vi "UHR-Fleezers Control (host) -Leonardo 04-2018 V3.vi"(0 "Tab Control":T5(tab)=enum."Trap Control (RF)") -> ()   [LabVIEW 2013] (continued)
      tunnel: w2352 -> [_ w2837]
      tunnel: w2351 -> [_ w2810]
      frame False {
      }
      frame True {
        w2817 = u32 0 items=["Horizontal", "Vertical", "Central", "1st Diagonal", "2nd Diagonal"] ("Type of Symmetry")
        w2845 = u32 0 items=["Horizontal", "Vertical", "Central", "1st Diagonal", "2nd Diagonal"] ("Type of Symmetry")
        w2848 = u32 0 items=["Horizontal", "Vertical", "Central", "1st Diagonal", "2nd Diagonal"] ("Type of Symmetry")
        w2877 = u32 0 items=["Horizontal", "Vertical", "Central", "1st Diagonal", "2nd Diagonal"] ("Type of Symmetry")
        n1850 = Index Array(array=w2906, index=10) -> (element=w2912:waveform(dbl))
        n1851 = Index Array(array=w2906, index=11) -> (element=w2909:waveform(dbl))
        n1852 = local read "Cycles/step (MCL)"() -> (w2862:u64)
        n1853 = Index Array(array=w2906, index="Channel") -> (element=w2908:waveform(dbl))
        n1854 = Unbundle(w2810) -> ("New Image"=w2809:T3, "New Image"=w2808:T3, "New Image"=w2807:T3, "New Image"=w2806:T3)
        n1855 = Unbundle By Name(w2912) -> ("Y"=w2864:dbl[])
        n1856 = Unbundle By Name(w2909) -> ("Y"=w2866:dbl[])
        n1857 = Unbundle By Name(w2908) -> ("Y"=w2871:dbl[])
        n1858 = call "downsample 1D array - double.vi"("Ave N"=w2862, "Array In"=w2864) -> ("Array Out"=w2863:dbl[])  [unwired: 1 out]
        n1859 = call "downsample 1D array - double.vi"("Ave N"=w2862, "Array In"=w2866) -> ("Array Out"=w2865:dbl[])  [unwired: 1 out]
        n1860 = call "downsample 1D array - double.vi"("Ave N"=w2862, "Array In"=w2871) -> ("Array Out"=w2870:dbl[])  [unwired: 1 out]
        n1861 = feedback #12(w2932) -> (w2933:dbl[])
        n1862 = Build Array (concatenate)(w2933, w2932) -> (w2914:dbl[])
        n1863 = feedback #13(w2837) -> (w2839:dbl[])
        n1864 = Build Array (concatenate)(w2839, w2837) -> (w2838:dbl[])
        n1865 = local read "Scan steps (MCL)"() -> (w2819:u64)
        n1866 = Select(t=w2932, s=w2836, f=w2914) -> (s? t:f=w2918:dbl[])
        n1867 = feedback-in #12(w2918) -> ()
        n1868 = Select(t=w2837, s=w2836, f=w2838) -> (s? t:f=w2820:dbl[])
        n1869 = feedback-in #13(w2820) -> ()
        n1870 = local read "Scan lines (y)"() -> (w2805:u64)
        n1871 = local read "N APD Samp/step"() -> (w2821:dbl)
        n1872 = feedback #14(w2863) -> (w2920:dbl[])
        n1873 = Build Array (concatenate)(w2920, w2863) -> (w2911:dbl[])
        n1874 = feedback #15(w2870) -> (w2930:dbl[])
        n1875 = Build Array (concatenate)(w2930, w2870) -> (w2929:dbl[])
        n1876 = feedback #16(w2865) -> (w2922:dbl[])
        n1877 = Build Array (concatenate)(w2922, w2865) -> (w2923:dbl[])
        n1878 = Select(t=w2863, s=w2836, f=w2911) -> (s? t:f=w2867:dbl[])
        n1879 = feedback-in #14(w2867) -> ()
        n1880 = Select(t=w2870, s=w2836, f=w2929) -> (s? t:f=w2869:dbl[])
        n1881 = feedback-in #15(w2869) -> ()
        n1882 = Select(t=w2865, s=w2836, f=w2923) -> (s? t:f=w2868:dbl[])
        n1883 = feedback-in #16(w2868) -> ()
        n1884 = Multiply(x=w2819, y=u64 2) -> (x*y=w2804:u64)
        n1885 = call "integrate 1D array interval - double.vi"("Ave N"=w2821, "Array In"=w2820) -> ("Array Out"=w2832:dbl[])  [unwired: 1 out]
        n1886 = call "integrate 1D array interval - double.vi"("Ave N"=w2821, "Array In"=w2918) -> ("Array Out"=w2917:dbl[])  [unwired: 1 out]
        n1887 = Array Size(array=w2832) -> (size(s)=w2833:i32)
        n1888 = Array Size(array=w2917) -> (size(s)=w2919:i32)
        n1889 = Multiply(x=w2805, y=w2804) -> (x*y=w2835:u64)
        n1890 = Multiply(x=w2805, y=w2804) -> (x*y=w2927:u64)
        n1891 = call-poly <vilib>:"Mean.vi"("X"=w2867) -> ("mean"=w2851:dbl)  [unwired: 1 out]
        n1892 = Subtract(x=w2835, y=w2833) -> (x-y=w2826:u64)
        n1893 = call-poly <vilib>:"Mean.vi"("X"=w2869) -> ("mean"=w2856:dbl)  [unwired: 1 out]
        n1894 = call-poly <vilib>:"Mean.vi"("X"=w2868) -> ("mean"=w2854:dbl)  [unwired: 1 out]
        n1895 = call-poly <vilib>:"Mean.vi"("X"=w2832) -> ("mean"=w2823:dbl)  [unwired: 1 out]
        n1896 = Subtract(x=w2927, y=w2919) -> (x-y=w2861:u64)
        n1897 = call-poly <vilib>:"Mean.vi"("X"=w2917) -> ("mean"=w2858:dbl)  [unwired: 1 out]
        n1898 = Initialize Array(1.0 ("element"), w2826) -> (w2822:dbl[])
        n1899 = Initialize Array(1.0 ("element"), w2861) -> (w2852:dbl[])
        n1900 = Multiply(x=w2822, y=w2823) -> (x*y=w2824:dbl[])
        n1901 = Multiply(x=w2852, y=w2854) -> (x*y=w2855:dbl[])
        n1902 = Multiply(x=w2852, y=w2856) -> (x*y=w2857:dbl[])
        n1903 = Multiply(x=w2852, y=w2851) -> (x*y=w2853:dbl[])
        n1904 = Multiply(x=w2852, y=w2858) -> (x*y=w2859:dbl[])
        n1905 = Build Array (concatenate)(w2867, w2853) -> (w2921:dbl[])
        n1906 = Build Array (concatenate)(w2869, w2857) -> (w2925:dbl[])
        n1907 = Build Array (concatenate)(w2868, w2855) -> (w2924:dbl[])
        n1908 = Build Array (concatenate)(w2832, w2824) -> (w2834:dbl[])
        n1909 = Build Array (concatenate)(w2917, w2859) -> (w2926:dbl[])
        n1910 = Reshape Array(w2921, w2805, w2804) -> (w2887:dbl[][])
        n1911 = Reshape Array(w2834, w2805, w2804) -> (w2830:dbl[][])
        n1912 = Reshape Array(w2925, w2805, w2804) -> (w2879:dbl[][])
        n1913 = Reshape Array(w2924, w2805, w2804) -> (w2894:dbl[][])
        n1914 = Reshape Array(w2926, w2805, w2804) -> (w2904:dbl[][])
        n1915 = Array Subset(array=w2894, index (col)=0 ("index"), length (col)=w2819) -> (w2899:dbl[][])  [unwired: 2 in]
        n1916 = Array Subset(array=w2894, index (col)=w2819) -> (w2897:dbl[][])  [unwired: 3 in]
        n1917 = Array Subset(array=w2879, index (col)=0 ("index"), length (col)=w2819) -> (w2885:dbl[][])  [unwired: 2 in]
        n1918 = Array Subset(array=w2879, index (col)=w2819) -> (w2883:dbl[][])  [unwired: 3 in]
        n1919 = Array Subset(array=w2830, index (col)=0 ("index"), length (col)=w2819) -> (w2829:dbl[][])  [unwired: 2 in]
        n1920 = Array Subset(array=w2830, index (col)=w2819) -> (w2827:dbl[][])  [unwired: 3 in]
        n1921 = Array Subset(array=w2904, index (col)=0 ("index"), length (col)=w2819) -> (w2903:dbl[][])  [unwired: 2 in]
        n1922 = Array Subset(array=w2904, index (col)=w2819) -> (w2901:dbl[][])  [unwired: 3 in]
        n1923 = Array Subset(array=w2887, index (col)=0 ("index"), length (col)=w2819) -> (w2892:dbl[][])  [unwired: 2 in]
        n1924 = Array Subset(array=w2887, index (col)=w2819) -> (w2890:dbl[][])  [unwired: 3 in]
        n1925 = for {
          tunnel: w2899 -> [w2941] mode=indexing
          tunnel: [w2940] -> w2898 mode=indexing
          workers-P: _ -> [_]
          n1926 = Reverse 1D Array(array=w2941) -> (reversed array=w2940:dbl[])
        }
        n1927 = for {
          tunnel: w2885 -> [w2937] mode=indexing
          tunnel: [w2936] -> w2884 mode=indexing
          workers-P: _ -> [_]
          n1928 = Reverse 1D Array(array=w2937) -> (reversed array=w2936:dbl[])
        }
        n1929 = for {
          tunnel: w2829 -> [w2935] mode=indexing
          tunnel: [w2934] -> w2828 mode=indexing
          workers-P: _ -> [_]
          n1930 = Reverse 1D Array(array=w2935) -> (reversed array=w2934:dbl[])
        }
        n1931 = for {
          tunnel: w2903 -> [w2943] mode=indexing
          tunnel: [w2942] -> w2902 mode=indexing
          workers-P: _ -> [_]
          n1932 = Reverse 1D Array(array=w2943) -> (reversed array=w2942:dbl[])
        }
        n1933 = for {
          tunnel: w2892 -> [w2939] mode=indexing
          tunnel: [w2938] -> w2891 mode=indexing
          workers-P: _ -> [_]
          n1934 = Reverse 1D Array(array=w2939) -> (reversed array=w2938:dbl[])
        }
        n1935 = Index Array(array=w2904, index (row)=0) -> (element=→"Waveform Graph":dbl[])  [unwired: 1 in]
        n1936 = Add(x=w2898, y=w2897) -> (x+y=w2896:dbl[][])
        n1937 = Add(x=w2884, y=w2883) -> (x+y=w2882:dbl[][])
        n1938 = Add(x=w2828, y=w2827) -> (x+y=w2812:dbl[][])
        n1939 = Add(x=w2902, y=w2901) -> (x+y=w2876:dbl[][])
        n1940 = Add(x=w2891, y=w2890) -> (x+y=w2889:dbl[][])
        n1941 = Divide(x=w2882, y=2) -> (x/y=w2880:dbl[][])
        n1942 = Divide(x=w2896, y=2) -> (x/y=w2841:dbl[][])
        n1943 = Divide(x=w2889, y=2) -> (x/y=w2843:dbl[][])
        n1944 = To Single Precision Float(number=w2876) -> (single precision float=w2875:sgl[][])
        n1945 = Transpose 2D Array(2D array=w2880) -> (transposed array=→"Data map":dbl[][])
        n1946 = To Single Precision Float(number=w2812) -> (single precision float=w2816:sgl[][])
        n1947 = To Single Precision Float(number=w2841) -> (single precision float=w2847:sgl[][])
        n1948 = To Single Precision Float(number=w2843) -> (single precision float=w2844:sgl[][])
        n1949 = call "IMAQ ArrayToImage"("Image Pixels (Float)"=w2875, "Image"=w2809) -> ("Image Out"=w2878:T3)  [unwired: 8 in, 1 out]
        n1950 = call "IMAQ ArrayToImage"("Image Pixels (Float)"=w2816, "Image"=w2808) -> ("Image Out"=w2818:T3)  [unwired: 8 in, 1 out]
        n1951 = call "IMAQ ArrayToImage"("Image Pixels (Float)"=w2847, "Image"=w2807) -> ("Image Out"=w2849:T3)  [unwired: 8 in, 1 out]
        n1952 = call "IMAQ ArrayToImage"("Image Pixels (Float)"=w2844, "Image"=w2806) -> ("Image Out"=w2846:T3)  [unwired: 8 in, 1 out]
        n1953 = call "IMAQ Symmetry"("Type of Symmetry"=w2877, "Image Src"=w2878) -> ("Image Dst Out"=w2873:T3)  [unwired: 3 in, 1 out]
        n1954 = call "IMAQ Symmetry"("Type of Symmetry"=w2817, "Image Src"=w2818) -> ("Image Dst Out"=w2814:T3)  [unwired: 3 in, 1 out]
        n1955 = call "IMAQ Symmetry"("Type of Symmetry"=w2848, "Image Src"=w2849) -> ("Image Dst Out"=→"Detection Laser X":T3)  [unwired: 3 in, 1 out]
        n1956 = call "IMAQ Symmetry"("Type of Symmetry"=w2845, "Image Src"=w2846) -> ("Image Dst Out"=→"Detection Laser Y":T3)  [unwired: 3 in, 1 out]
        n1957 = call "IMAQ Set Simple Calibration"("Calibration Axis Info"=T37 {"Origin Pixel"={"X"=0.0, "Y"=0.0}, "Angle Relative to Horizontal (deg)"=0.0, "Axis Reference"=0}, "Grid Descriptor"=T38 {"X Step"=0.3, "Y Step"=0.3, "Unit"=enum."Undefined"}, "Image"=w2873) -> ("Calibrated Image"=→"APD 1":T3)  [unwired: 7 in, 1 out]
        n1958 = call "IMAQ Set Simple Calibration"("Calibration Axis Info"=T37 {"Origin Pixel"={"X"=0.0, "Y"=0.0}, "Angle Relative to Horizontal (deg)"=0.0, "Axis Reference"=0}, "Grid Descriptor"=T38 {"X Step"=0.3, "Y Step"=0.3, "Unit"=enum."Undefined"}, "Image"=w2814) -> ("Calibrated Image"=→"APD 2":T3)  [unwired: 7 in, 1 out]
      }
    }
    n1959 = Subtract(x=w2358, y="APD 2 Offset") -> (x-y=w2355:waveform(dbl))
    n1960 = Subtract(x=w2360, y="APD 1 Offset") -> (x-y=w2356:waveform(dbl))
    n1961 = Index Array(array=w2375, index=3) -> (element=w2434:waveform(dbl))
    n1962 = Index Array(array=w2375, index=6) -> (element=w2431:waveform(dbl))
    n1963 = Build Array(w2356, w2355) -> (→"APD Chart":waveform(dbl)[])
    n1964 = Array Size(array=w2424) -> (size(s)=w2472:i32)
    n1965 = call <vilib>:"Std Deviation and Variance.vi"("X"=w2368) -> ("standard deviation"=w2367:dbl)  [unwired: 1 in, 2 out]
    n1966 = Add Array Elements(numeric array=w2368) -> (sum=w2370:u32)
    n1967 = Add Array Elements(numeric array=w2424) -> (sum=w2482:u32)
    n1968 = call <vilib>:"Std Deviation and Variance.vi"("X"=w2424) -> ("standard deviation"=w2423:dbl)  [unwired: 1 in, 2 out]
    n1969 = Divide(x=w2367, y=w2366) -> (x/y=w2363:dbl)
    "Rate sigma (Hz) 2" <- w2363
    n1970 = Multiply(x=w2366, y=w2472) -> (x*y=w2369:dbl)
    "Int. Time (s)" <- w2369
    n1971 = Divide(x=w2370, y=w2369) -> (x/y=w2364:dbl)
    "APD 2 Rate (Hz)" <- w2364
    n1972 = Divide(x=w2482, y=w2369) -> (x/y=w2421:dbl)
    "APD 1 Rate (Hz)" <- w2421
    n1973 = Divide(x=w2423, y=w2366) -> (x/y=w2422:dbl)
    "Rate sigma (Hz)" <- w2422
    n1974 = Divide(x=w2363, y=w2364) -> (x/y=→"Sigma/Mean 2":dbl)
    n1975 = Divide(x=w2422, y=w2421) -> (x/y=→"Sigma/Mean":dbl)
    n1976 = case shown="2" "Calibration" {
      tunnel: "T1 alpha_x (nm/V)" -> [_ w2772 w2793]
      tunnel: "T1 kappa_x (pN/nm)" -> [_ _ w2783]
      tunnel: "T2 alpha_x (nm/V)" -> [_ w2771 w2791]
      tunnel: "T2 kappa_x (pN/nm)" -> [_ _ w2784]
      tunnel: w2434 -> [w2754 w2769 w2789]
      tunnel: w2431 -> [w2753 w2767 w2787]
      tunnel: [w2754 w2766 w2786] -> w2224
      tunnel: [w2753 w2765 w2785] -> w2230
      tunnel: ["T1 X (V)" ("Label.Text") "T1 X (nm)" ("Label.Text") "T1 X (pN)" ("Label.Text")] -> w2452
      tunnel: ["T2 X (V)" ("Label.Text") "T2 X (nm)" ("Label.Text") "T2 X (pN)" ("Label.Text")] -> w2451
      tunnel: ["Position (V)" ("Label.Text") "Position (nm)" ("Label.Text") "Force (pN)" ("Label.Text")] -> w2453
      tunnel: w2433 -> [_ w2757 w2776]
      tunnel: w2435 -> [_ w2760 w2778]
      tunnel: ["Mean (V)" ("Label.Text") "Mean (nm)" ("Label.Text") "Mean (pN)" ("Label.Text")] -> w2448
      tunnel: ["Difference (V)" ("Label.Text") "Difference (nm)" ("Label.Text") "Difference (pN)" ("Label.Text")] -> w2383
      frame 0, Default {
      }
      frame 1 {
        # "position"
        n1977 = Unbundle By Name(w2769) -> ("Y"=w2773:dbl[])
        n1978 = Unbundle By Name(w2767) -> ("Y"=w2758:dbl[])
        n1979 = Subtract(x=w2773, y=w2760) -> (x-y=w2761:dbl[])
        n1980 = Subtract(x=w2758, y=w2757) -> (x-y=w2759:dbl[])
        n1981 = Multiply(x=w2759, y=w2771) -> (x*y=w2768:dbl[])
        n1982 = Multiply(x=w2772, y=w2761) -> (x*y=w2770:dbl[])
        n1983 = Bundle By Name(cluster=w2767, "Y"=w2768) -> (w2765:waveform(dbl))
        n1984 = Bundle By Name(cluster=w2769, "Y"=w2770) -> (w2766:waveform(dbl))
      }
      frame 2 {
        # "force"
        n1985 = Unbundle By Name(w2789) -> ("Y"=w2794:dbl[])
        n1986 = Unbundle By Name(w2787) -> ("Y"=w2792:dbl[])
        n1987 = Subtract(x=w2792, y=w2776) -> (x-y=w2777:dbl[])
        n1988 = Subtract(x=w2794, y=w2778) -> (x-y=w2779:dbl[])
        n1989 = Compound Arithmetic op=MULTIPLY(w2777, w2791, w2784) -> (w2788:dbl[])
        n1990 = Compound Arithmetic op=MULTIPLY(w2783, w2793, w2779) -> (w2790:dbl[])
        n1991 = Bundle By Name(cluster=w2787, "Y"=w2788) -> (w2785:waveform(dbl))
        n1992 = Bundle By Name(cluster=w2789, "Y"=w2790) -> (w2786:waveform(dbl))
      }
    }
    n1993 = feedback-in #17("Calibration") -> ()
    n1994 = feedback #17(u16 1 ("Calibration")) -> (w2455:u16)
    n1995 = local read "Trap 2 Bead Size (nm)"() -> (w2263:dbl)
    n1996 = local read "Trap 1 Bead Size (nm)"() -> (w2262:dbl)
    n1997 = local read "AOM X Cal (nm/MHz)"() -> (w2260:dbl)
    n1998 = local read "Trap Delta (MHz)"() -> (w2259:dbl)
    n1999 = Not Equal?(x=w2455, y="Calibration") -> (x != y?=w2412:bool)
    n2000 = Multiply(x=w2260, y=w2259) -> (x*y=w2264:dbl)
    n2001 = Unbundle By Name(w2224) -> ("Y"=w2229:dbl[])
    n2002 = Unbundle By Name(w2230) -> ("Y"=w2228:dbl[])
    n2003 = Add(x=w2263, y=w2262) -> (x+y=w2266:dbl)
    n2004 = case shown="False" "Negate trap 2 force" {
      tunnel: [-1.0 1.0] -> w2441
      frame False {
      }
      frame True {
      }
    }
    n2005 = Unbundle By Name(w2434) -> ("Y"=w2437:dbl[])
    n2006 = Unbundle By Name(w2431) -> ("Y"=w2440:dbl[])
    n2007 = Divide(x=w2266, y=2.0) -> (x/y=w2261:dbl)
    n2008 = Subtract(x=w2229, y=w2228) -> (x-y=w2226:dbl[])
    n2009 = Subtract(x=w2437, y=w2435) -> (x-y=w2438:dbl[])
    n2010 = Subtract(x=w2440, y=w2433) -> (x-y=w2439:dbl[])
    n2011 = Divide(x=w2226, y=2.0) -> (x/y=w2225:dbl[])
    n2012 = Multiply(x=w2439, y="T2 alpha_x (nm/V)") -> (x*y=w2430:dbl[])
    n2013 = Multiply(x="T1 alpha_x (nm/V)", y=w2438) -> (x*y=w2429:dbl[])
    n2014 = Multiply(x=w2230, y=w2441) -> (x*y=w2442:waveform(dbl))
    n2015 = Bundle By Name(cluster=w2224, "Y"=w2225) -> (w2223:waveform(dbl))
    n2016 = case shown="True" "Read Lateness and Rel Phase" {
      tunnel: w2236 -> [w2720 w2742]
      tunnel: w2275 -> [w2721 w2741]
      tunnel: [w2720 w2740] -> w2427
      tunnel: [w2721 w2739] -> w2426
      frame False {
      }
      frame True {
        n2017 = xnode "Read/Write Control"("FPGA VI Reference In"=w2742, "error in"=w2741) -> ("FPGA VI Reference Out"=w2740:T20, "error out"=w2739:errorcluster, "GI Relative phase"=→"GI relative phase":i16, "Relative phase"=→"Relative phase (AI1)":i16, "AI Late Counter"=→"Late Counter (AI1)":u8, "GI Late Counter"=→"GI Late Counter":u8, "MCL Late Counter"=→"MCL Late Counter":u8, "MCL Relative Phase"=→"Relative Phase (MCL)":i16, "APD Acq Relative Phase"=→"APD Acq Relative Phase":i16, "APD 1 Gate Relative Phase"=→"APD 1 Gate Relative Phase":i16, "APD 2 Gate Relative Phase"=→"APD 2 Gate Relative Phase":i16, "APD Acq Late Counter"=→"APD Acq Late Counter":u16, "APD 1 Gate Late Counter"=→"APD 1 Gate Late Counter":u8, "APD 2 Gate Late Counter"=→"APD 2 Gate Late Counter":u8, "Green FB Relative Phase"=→"Relative phase (Green FB)":i16, "GI Relative phase"=→"GI relative phase 2":i16, "GI Late Counter 2"=→"GI Late Counter 2":u16, "Trap Pos FIFO Timeout"=→"Trap Pos FIFO Timeout":u16, "Trap AI FIFO Timeout"=→"Trap AI FIFO Timeout":u16)
      }
    }
    n2018 = Subtract(x=w2430, y=w2429) -> (x-y=w2258:dbl[])
    n2019 = call-poly <vilib>:"Mean.vi"("X"=w2258) -> ("mean"=w2265:dbl)  [unwired: 1 out]
    n2020 = Add(x=w2264, y=w2265) -> (x+y=w2268:dbl)
    n2021 = Subtract(x=w2268, y=w2261) -> (x-y=→"Tether Extension (nm, calculated)":dbl)
    n2022 = Unbundle By Name(w2230) -> ("Y"=w2221:dbl[])
    n2023 = Unbundle By Name(w2224) -> ("Y"=w2222:dbl[])
    n2024 = Build Array(w2224, w2442, w2223) -> (→"Force":waveform(dbl)[])
    n2025 = Subtract(x=w2258, y="Offset (nm)") -> (x-y=w2402:dbl[])
    n2026 = call-poly <vilib>:"Mean.vi"("X"=w2221) -> ("mean"=w2219:dbl)  [unwired: 1 out]
    "T2 X" <- w2219
    n2027 = call-poly <vilib>:"Mean.vi"("X"=w2222) -> ("mean"=w2220:dbl)  [unwired: 1 out]
    "T1 X" <- w2220
    n2028 = Subtract(x=w2222, y=w2221) -> (x-y=w2404:dbl[])
    n2029 = Bundle By Name(cluster=w2434, "Y"=w2402) -> (w2374:waveform(dbl))
    "Bead Separation" <- w2374
    n2030 = Divide(x=w2404, y=2.0) -> (x/y=→"Vec Mean of T1 T2":dbl[])
    n2031 = case shown="True" w2412 {
      tunnel: w2453 -> [_ w2747]
      tunnel: w2452 -> [_ w2746]
      tunnel: w2451 -> [_ w2745]
      tunnel: w2448 -> [_ w2744]
      tunnel: w2383 -> [_ w2743]
      frame False {
      }
      frame True {
        n2032 = property on="Force" class="WFChart (strict)"("YScale.NameLbl.Text"=w2747) -> ()  [unwired: 2 in, 2 out]
        n2033 = property on="T2 X" class="DigNum (strict)"("Caption.Text"=w2745) -> ()  [unwired: 2 in, 2 out]
        n2034 = property on="T1 X" class="DigNum (strict)"("Caption.Text"=w2746) -> ()  [unwired: 2 in, 2 out]
        n2035 = property on="Mean" class="DigNum (strict)"("Caption.Text"=w2744) -> ()  [unwired: 2 in, 2 out]
        n2036 = property on="Difference" class="DigNum (strict)"("Caption.Text"=w2743) -> ()  [unwired: 2 in, 2 out]
      }
    }
    n2037 = local read "Tether"() -> (w2406:bool)
    n2038 = Subtract(x=w2220, y=w2219) -> (x-y=w2450:dbl)
    n2039 = Add(x=w2220, y=w2219) -> (x+y=→"Difference":dbl)
    n2040 = feedback #18(w2402) -> (w2401:dbl[])
    n2041 = Divide(x=w2450, y=2.0) -> (x/y=w2233:dbl)
    "Mean" <- w2233
    n2042 = case shown="True" w2406 {
      tunnel: w2233 -> [_ w2679]
      frame False {
      }
      frame True {
        n2043 = Greater?(x="Lost Tether Alarm Threshold (pN)", y=w2679) -> (0:w2677:bool)
        n2044 = case shown="True" w2677 {
          frame False {
          }
          frame True {
            n2045 = flat-sequence {
              frame #0 {
                # "stop only if saving"
                n2046 = local read "Saving..."() -> (w2692:bool)
                n2047 = And(x=w2692, y="TA Cancel Save?") -> (x .and. y?=w2691:bool)
                n2048 = local write "Stop Saving"(w2691) -> ()
              }
              frame #1 {
                n2049 = case shown="True" "TA Green Off?" {
                  frame False {
                  }
                  frame True {
                    w2695 = FALSE ("Fl. Triggered...")
                    n2050 = local write "Fl. Triggered..."(w2695) -> ()
                    n2051 = property on="Green Laser ON/Interlacing" class="Bool (strict)"("Val(Sgnl)"=w2695) -> ()  [unwired: 2 in, 2 out]
                  }
                }
              }
            }
            n2052 = local read "Time tether formed"() -> (w2686:timestamp)
            n2053 = Get Date/Time In Seconds() -> (seconds since 1Jan1904=w2687:timestamp)
            n2054 = Subtract(x=w2687, y=w2686) -> (x-y=w2685:dbl)
            n2055 = Number To Decimal String(number=w2685) -> (decimal integer string=w2682:string)  [unwired: 1 out]
            n2056 = local read "Messages"() -> (w2689:string)
            n2057 = call <vilib>:"Beep.vi"() -> ()  [unwired: 3 in, 9 out]
            n2058 = Concatenate Strings("Lost tether (" ("Message to add"), w2682, " s)." ("string")) -> (w2684:string)
            n2059 = local write "Tether"(FALSE ("Tether")) -> ()
            n2060 = call "Update messages.vi"("Message to add"=w2684, "Old message string"=w2689) -> ("New message string"=w2688:string)
            n2061 = local write "Messages"(w2688) -> ()
            n2062 = property on="Trap Pos. FB ON" class="Bool (strict)"("Val(Sgnl)"=FALSE ("Value (Signaling)")) -> ()  [unwired: 2 in, 2 out]
          }
        }
      }
    }
    n2063 = Build Array (concatenate)(w2402, w2401) -> (w2400:dbl[])
    n2064 = Split 1D Array(array=w2400, index=w2286) -> (first subarray=w2396:dbl[])  [unwired: 1 out]
    n2065 = feedback-in #18(w2396) -> ()
    n2066 = call-poly <vilib>:"Mean.vi"("X"=w2396) -> ("mean"=w2395:dbl)  [unwired: 1 out]
    "Bead Mean (nm)" <- w2395
    n2067 = Subtract(x=w2396, y=w2395) -> (x-y=w2394:dbl[])
    n2068 = Square(x=w2394) -> (x^2=w2393:dbl[])
    n2069 = case shown="True" "Semi Passive ON" {
      tunnel: "Semi Passive mode" -> [_ w2560]
      tunnel: "Jump Force (pN)" -> [_ w2559]
      tunnel: w2233 -> [_ w2558]
      frame False {
      }
      frame True {
        n2070 = case shown="\"Use Feedback\"" w2560 {
          tunnel: w2559 -> [_ w2563 w2579]
          tunnel: w2558 -> [_ w2562 w2578]
          frame "None" {
          }
          frame "Use Feedback" {
            n2071 = local read "Target Force (pN)"() -> (w2565:dbl)
            n2072 = Less?(x=w2563, y=w2565) -> (x < y?=w2564:bool)
            n2073 = case shown="True" w2564 {
              tunnel: w2563 -> [w2572 w2575]
              tunnel: w2562 -> [w2571 w2574]
              tunnel: [w2570 w2573] -> w2561
              frame False {
                n2074 = Less?(x=w2572, y=w2571) -> (x < y?=w2570:bool)
              }
              frame True {
                n2075 = Greater?(x=w2575, y=w2574) -> (0:w2573:bool)
              }
            }
            n2076 = case shown="True" w2561 {
              frame False {
                n2077 = local read "Trap Pos. FB ON"() -> (w2566:bool)
                n2078 = case shown="True" w2566 {
                  frame False {
                  }
                  frame True {
                    n2079 = property on="Trap Pos. FB ON" class="Bool (strict)"("Val(Sgnl)"=FALSE) -> ()  [unwired: 2 in, 2 out]
                  }
                }
              }
              frame True {
                n2080 = local read "Trap Pos. FB ON"() -> (w2568:bool)
                n2081 = case shown="False" w2568 {
                  frame False {
                    n2082 = property on="Trap Pos. FB ON" class="Bool (strict)"("Val(Sgnl)"=TRUE) -> ()  [unwired: 2 in, 2 out]
                  }
                  frame True {
                  }
                }
              }
            }
          }
          frame "Sharp Jump" {
            n2083 = local read "Target Force (pN)"() -> (w2581:dbl)
            n2084 = Greater?(x=w2579, y=w2581) -> (0:w2580:bool)
            n2085 = case shown="True" w2580 {
              tunnel: w2579 -> [w2596 w2600]
              tunnel: w2578 -> [w2597 w2599]
              tunnel: [w2595 w2598] -> w2577
              frame False {
                n2086 = Greater?(x=w2597, y=w2596) -> (0:w2595:bool)
              }
              frame True {
                n2087 = Less?(x=w2600, y=w2599) -> (x < y?=w2598:bool)
              }
            }
            n2088 = Subtract(x=w2579, y=w2581) -> (x-y=w2576:dbl)
            n2089 = case shown="True" w2577 {
              tunnel: w2576 -> [_ w2587]
              frame False {
              }
              frame True {
                n2090 = local read "T1 kappa_x (pN/nm)"() -> (w2592:dbl)
                n2091 = local read "T2 kappa_x (pN/nm)"() -> (w2593:dbl)
                n2092 = Reciprocal(x="DNA stiffness (pN / nm)") -> (1/x=w2589:dbl)
                n2093 = Reciprocal(x=w2592) -> (1/x=w2591:dbl)
                n2094 = Reciprocal(x=w2593) -> (1/x=w2590:dbl)
                n2095 = Compound Arithmetic op=ADD(w2591, w2590, w2589) -> (w2588:dbl)
                n2096 = local read "AOM X Cal (nm/MHz)"() -> (w2586:dbl)
                n2097 = Multiply(x=w2588, y=w2587) -> (x*y=w2585:dbl)
                n2098 = local read "Trap Delta (MHz)"() -> (w2583:dbl)
                n2099 = Divide(x=w2585, y=w2586) -> (x/y=w2584:dbl)
                n2100 = Subtract(x=w2583, y=w2584) -> (x-y=w2582:dbl)
                n2101 = property on="Trap Delta (MHz)" class="DigNum (strict)"("Val(Sgnl)"=w2582) -> ()  [unwired: 2 in, 2 out]
              }
            }
          }
        }
      }
    }
    n2102 = call-poly <vilib>:"Mean.vi"("X"=w2393) -> ("mean"=w2392:dbl)  [unwired: 1 out]
    n2103 = Square Root(x=w2392) -> (sqrt(x)=w2391:dbl)
    n2104 = Multiply(x=10.0, y=w2391) -> (x*y=→"RMS (Ang)":dbl)
    n2105 = xnode "Read/Write Control"("FPGA VI Reference In"=w2427, "error in"=w2426) -> ("FPGA VI Reference Out"=w2536:T20, "error out"=w2530:errorcluster, "AI2 Y Sum Set 1"=w2526:i16, "AI2 Y Sum Set 2"=w2525:i16, "AI1 X Set 1"=w2320:fxp<+/-,16,1>, "AI1 X Set 2"=w2319:fxp<+/-,16,1>, "Trap Pos FB Int Signal"=→"Trap Pos FB Int Signal":fxp<+/-,24,9>, "Trap Pos FB Int-Norm Signal"=→"Trap Pos FB Int-Norm Signal":fxp<+/-,16,1>, "Trap Pos FB Action"=w2313:i64, "Scanning"=→"AOD Scanning":bool, "Scan I"=→"AOD Scan I":u64, "Scanning MCL"=w2528:bool, "Scan I (MCL)"=→"MCL Scan I":u64, "Green FB Signals"=w2467:T48, "BD1 amplitude 1 out"=w2218:u16, "BD1 amplitude 2 out"=w2203:u16)  [unwired: 1 out]
    "MCL Scanning" <- w2528
    "Trap Pos FB Action" <- w2313
    n2106 = local read "AI2 (V)"() -> (w2527:cluster{"Set 1":dbl, "Set 2":dbl})
    n2107 = Bundle By Name(cluster=w2527, "Set 1"=w2526, "Set 2"=w2525) -> (w2523:cluster{"Set 1":dbl, "Set 2":dbl})
    n2108 = Divide(x=w2313, y=327.67) -> (x/y=→"Action (%)":dbl)
    n2109 = local read "Trap X (AI1)"() -> (w2333:T1)
    n2110 = Divide(x=w2523, y=3276.7) -> (x/y=w2522:cluster{"Set 1":dbl, "Set 2":dbl})
    n2111 = local write "AI2 (V)"(w2522) -> ()
    n2112 = Bundle(cluster=w2333, "Trap 1"=w2320, "Trap 2"=w2319) -> (→"Trap X (AI1)":T1)
    n2113 = Scale By Power Of 2(n=i16 12, x=ext 1.0) -> (x*2^n=w2214:ext)
    n2114 = Subtract(x=w2214, y=ext 1.0) -> (x-y=w2211:ext)
    n2115 = Divide(x=w2467, y=3276.7) -> (x/y=w2463:T49)
    n2116 = Multiply(x=w2218, y=ext 100.0) -> (x*y=w2212:ext)
    n2117 = Unbundle By Name(w2463) -> ("Green FB Ch 0"=w2466:dbl, "Green FB Ch 1"=w2465:dbl, "Green FB Ch 2"=w2464:dbl)
    n2118 = local read "All FB On/Off"() -> (w2202:bool)
    n2119 = Divide(x=w2212, y=w2211) -> (x/y=w2201:ext)
    "Trap 1 amplitude" <- w2201
    n2120 = Scale By Power Of 2(n=i16 12, x=ext 1.0) -> (x*2^n=w2207:ext)
    n2121 = Subtract(x=w2207, y=ext 1.0) -> (x-y=w2210:ext)
    n2122 = Multiply(x=w2203, y=ext 100.0) -> (x*y=w2209:ext)
    n2123 = Divide(x=w2466, y=w2464) -> (x/y=w2462:dbl)
    n2124 = Divide(x=w2465, y=w2464) -> (x/y=w2461:dbl)
    n2125 = flat-sequence "To save data" {
      tunnel: [w3576] -> w2547
      tunnel: [w3577] -> w2546
      tunnel: w2498 -> [w3570]
      tunnel: w2398 -> [w3574]
      tunnel: ["Save Calibration"] -> w2519
      tunnel: w2516 -> [w3573]
      tunnel: [w3566] -> w2515
      tunnel: [w3563] -> w2514
      tunnel: [w3560] -> w2513
      tunnel: w2497 -> [w3562]
      tunnel: w2410 -> [w3556]
      tunnel: [w3556] -> w2409
      tunnel: ["Start Saving"] -> w2376
      tunnel: [w3550] -> w2302
      tunnel: [w3549] -> w2301
      tunnel: w2547 -> [w3811]
      tunnel: w2546 -> [w3810]
      tunnel: w2303 -> [w3809]
      tunnel: w2519 -> [w3808]
      tunnel: w2515 -> [w3806]
      tunnel: w2514 -> [w3805]
      tunnel: w2513 -> [w3804]
      tunnel: w2385 -> [w3803]
      tunnel: w2419 -> [w3802]
      tunnel: w2409 -> [w3801]
      tunnel: w2376 -> [w3800]
      tunnel: w2374 -> [w3799]
      tunnel: w2350 -> [w3798]
      tunnel: w2302 -> [w3797]
      tunnel: w2301 -> [w3796]
      tunnel: w2300 -> [w3795]
      frame #0 {
        n2126 = Or(x="Save N Sets", y="Start Saving") -> (x .or. y?=w3557:bool)
        n2127 = To Double Precision Float(number=w3573) -> (double precision float=w3567:dbl)
        n2128 = Build Array(w3557, "Save Calibration", w3570, w3562) -> (w3572:bool[])
        n2129 = Compound Arithmetic op=OR("Save Calibration", w3570, w3557, w3562) -> (w3575:bool)
        n2130 = Boolean Array To Number(Boolean array=w3572) -> (number=w3569:u32)
        n2131 = feedback #19(FALSE ("Save APD Data\nwith Trap Data")) -> (w3551:bool)
        n2132 = feedback #20(refnum<k0> refnum) -> (w3578:refnum<file>)
        n2133 = feedback #21(refnum<k0> refnum) -> (w3553:refnum<file>)
        n2134 = feedback #22(FALSE ("Save APD Data\nwith Trap Data")) -> (w3561:bool)
        n2135 = feedback #23(refnum<k0> refnum) -> (w3564:refnum<file>)
        n2136 = feedback #24(0) -> (w3580:i32)
        n2137 = feedback #25() -> (w3568:u32)  [unwired: 1 out]
        n2138 = case shown="True" w3575 {
          tunnel: [w3587 1] -> w3576
          tunnel: w3580 -> [w3589 _]
          tunnel: [w3588 w3607] -> w3577
          tunnel: w3578 -> [w3588 _]
          tunnel: w3574 -> [_ w3627]
          tunnel: w3567 -> [_ w3625]
          tunnel: w3569 -> [_ w3628]
          tunnel: [w3586 w3606] -> w3566
          tunnel: w3568 -> [w3586 _]
          tunnel: [w3585 w3604] -> w3563
          tunnel: w3564 -> [w3585 _]
          tunnel: [w3584 w3603] -> w3560
          tunnel: w3561 -> [w3584 _]
          tunnel: "Start Saving" -> [_ w3601]
          tunnel: w3556 -> [_ w3600]
          tunnel: [w3583 w3591] -> w3549
          tunnel: w3553 -> [w3583 _]
          tunnel: [w3582 w3590] -> w3550
          tunnel: w3551 -> [w3582 _]
          frame False {
            n2139 = Increment(x=w3589) -> (x+1=w3587:i32)
          }
          frame True {
            w3597 = FALSE ("Start Saving")
            w3602 = 9.0  # File Version
            w3610 = FALSE ("prepend array or string size? (T)")
            w3608 = T30."big-endian, network order" ("byte order (0:big-endian, network order)")
            # "write file headers"
            n2140 = local read "BD 1 Frequency 1 (MHz)"() -> (w3624:dbl)
            n2141 = local read "BD 2 Frequency 1 (MHz)"() -> (w3623:dbl)
            n2142 = local read "BD 1 Frequency 2 (MHz)"() -> (w3622:dbl)
            n2143 = local read "BD 2 Frequency 2 (MHz)"() -> (w3621:dbl)
            n2144 = local read "BD 1 Frequency 3 (MHz)"() -> (w3620:dbl)
            n2145 = local read "BD 2 Frequency 3 (MHz)"() -> (w3619:dbl)
            n2146 = Array Size(array=w3600) -> (size(s)=w3599:i32)
            n2147 = To Double Precision Float(number=w3599) -> (double precision float=w3598:dbl)
            n2148 = local write "Save Calibration"(w3597) -> ()
            n2149 = local write "Start Saving"(w3597) -> ()
            n2150 = Build Array("Save APD Data\nwith Trap Data", "Save Trap Pos. Data") -> (w3594:bool[])
            n2151 = Boolean Array To Number(Boolean array=w3594) -> (number=w3593:u32)
            n2152 = Build Array(w3624, w3623, w3622, w3621, w3620, w3619) -> (w3618:dbl[])
            n2153 = case shown="4" w3628 {
              tunnel: w3627 -> [w3699 w3719 w3735 w3773]
              tunnel: w3598 -> [w3704 w3726 w3755 w3792]
              tunnel: w3625 -> [w3703 w3725 w3754 w3791]
              tunnel: [w3700 w3721 w3746 w3783] -> w3616
              tunnel: [w3691 "Cal sets to save" w3736 w3774] -> w3606
              tunnel: w3618 -> [w3701 w3722 w3748 w3785]
              tunnel: "Save APD Data\nwith Trap Data" -> [w3698 _ w3732 w3771]
              tunnel: [w3698 w3713 w3732 w3771] -> w3603
              tunnel: w3602 -> [w3694 w3714 w3730 w3769]
              tunnel: w3601 -> [w3693 _ _ _]
              tunnel: [w3684 w3713 w3729 w3759] -> w3590
              tunnel: "Save Trap Pos. Data" -> [w3684 _ w3729 w3759]
              tunnel: w3593 -> [w3683 _ w3728 w3758]
              frame 1, Default {
                # "timeseries"
                n2154 = case shown="True" "Profile" {
                  tunnel: [w3707 w3710] -> w3688
                  tunnel: [w3707 w3709] -> w3687
                  tunnel: [w3707 w3708] -> w3686
                  tunnel: [w3707 w3712] -> w3685
                  frame False {
                    w3707 = 0.0 ("f")
                  }
                  frame True {
                    n2155 = local read "Current Position"() -> (w3711:dbl[])
                    n2156 = local read "Y change (mm)"() -> (w3712:dbl)
                    n2157 = call "subVI_explode3array.vi"("Array"=w3711) -> ("x"=w3710:dbl, "y"=w3709:dbl, "z"=w3708:dbl)  [unwired: 12 in]
                  }
                }
                n2158 = local read "Save ave N"() -> (w3706:dbl)
                n2159 = Multiply(x=w3706, y=w3699) -> (x*y=w3705:dbl)
                n2160 = To Double Precision Float(number=w3683) -> (double precision float=w3697:dbl)
                n2161 = Build Array(w3694, w3699, w3705, w3704, w3703, 0.0 ("f")) -> (w3702:dbl[])
                n2162 = Build Array(w3697, w3688, w3687, w3686, w3685) -> (w3695:dbl[])
                n2163 = Select(t=u32 4000000000, s=w3693, f="N sets to save") -> (s? t:f=w3691:u32)
                n2164 = Build Array (concatenate)(w3702, w3701, w3695) -> (w3700:dbl[])
              }
              frame 2 {
                w3716 = 0.0 ("f")
                w3713 = FALSE ("Save APD Data\nwith Trap Data")
                # "calibration"
                n2165 = Boolean To (0,1)(Boolean=w3713) -> (0, 1=w3718:i16)
                n2166 = To Double Precision Float(number=w3718) -> (double precision float=w3717:dbl)
                n2167 = Build Array(w3717, w3716, w3716, w3716, w3716) -> (w3715:dbl[])
                n2168 = Build Array(w3714, w3719, w3719, w3726, w3725, 1.0 ("t")) -> (w3723:dbl[])
                n2169 = Build Array (concatenate)(w3723, w3722, w3715) -> (w3721:dbl[])
                "Calibrating Trap..." <- TRUE ("Calibrating...")
              }
              frame 4 {
                w3733 = 0.0 ("f")
                # "write file header for a trap \nraster scan"
                # "scan dir (x/y = 0/1)"
                # "cycles/step"
                # "n scans (f/b)"
                # "steps"
                # "freq. range"
                # "AOD raster scan"
                n2170 = local read "Number of F/B Scans (AOD)"() -> (w3740:u16)
                n2171 = local read "Cycles/step (AOD)"() -> (w3742:u64)
                n2172 = local read "Scan Range (MHz)"() -> (w3745:dbl)
                n2173 = local read "Scan steps (AOD)"() -> (w3744:u64)
                n2174 = local read "Scan BD"() -> (w3752:bool)
                n2175 = local read "Save ave N"() -> (w3757:dbl)
                n2176 = Boolean To (0,1)(Boolean=w3752) -> (0, 1=w3751:i16)
                n2177 = To Double Precision Float(number=w3740) -> (double precision float=w3739:dbl)
                n2178 = To Double Precision Float(number=w3744) -> (double precision float=w3743:dbl)
                n2179 = To Double Precision Float(number=w3742) -> (double precision float=w3741:dbl)
                n2180 = To Double Precision Float(number=w3751) -> (double precision float=w3750:dbl)
                n2181 = Multiply(x=w3757, y=w3735) -> (x*y=w3756:dbl)
                n2182 = To Double Precision Float(number=w3728) -> (double precision float=w3734:dbl)
                n2183 = Build Array(w3734, w3733, w3733, w3733, w3733) -> (w3731:dbl[])
                n2184 = local read "N sets should be saved"() -> (w3737:dbl)
                n2185 = Build Array(w3750, w3745, w3743, w3741, w3739) -> (w3747:dbl[])
                n2186 = Build Array(w3730, w3735, w3756, w3755, w3754, 2.0 ("t")) -> (w3749:dbl[])
                n2187 = Round Toward +Infinity(x=w3737) -> (ceil(x): smallest int >= x=w3738:dbl)
                n2188 = Build Array (concatenate)(w3749, w3748, w3731, w3747) -> (w3746:dbl[])
                n2189 = To Unsigned Long Integer(number=w3738) -> (unsigned 32bit integer=w3736:u32)
              }
              frame 8 {
                w3766 = 0.0 ("f")
                # "MCL raster scan"
                n2190 = local read "Number of scans (MCL)"() -> (w3761:u64)
                n2191 = local read "Scan lines (y)"() -> (w3760:u64)
                n2192 = local read "2D or 1D Scan"() -> (w3763:bool)
                n2193 = local read "Scan Range (V)\n(of steps)"() -> (w3782:dbl)
                n2194 = local read "Fast Scan Dir"() -> (w3789:bool)
                n2195 = local read "Cycles/step (MCL)"() -> (w3779:u64)
                n2196 = local read "Scan steps (MCL)"() -> (w3781:u64)
                n2197 = Select(t=w3760, s=w3763, f=w3761) -> (s? t:f=w3762:u64)
                n2198 = Boolean To (0,1)(Boolean=w3763) -> (0, 1=w3765:i16)
                n2199 = local read "Save ave N"() -> (w3794:dbl)
                n2200 = local read "Initial X"() -> (w3768:dbl)
                n2201 = local read "Initial Y"() -> (w3767:dbl)
                n2202 = To Double Precision Float(number=w3765) -> (double precision float=w3764:dbl)
                n2203 = Boolean To (0,1)(Boolean=w3789) -> (0, 1=w3788:i16)
                n2204 = To Double Precision Float(number=w3762) -> (double precision float=w3777:dbl)
                n2205 = To Double Precision Float(number=w3781) -> (double precision float=w3780:dbl)
                n2206 = To Double Precision Float(number=w3779) -> (double precision float=w3778:dbl)
                n2207 = To Double Precision Float(number=w3788) -> (double precision float=w3787:dbl)
                n2208 = Multiply(x=w3794, y=w3773) -> (x*y=w3793:dbl)
                n2209 = To Double Precision Float(number=w3758) -> (double precision float=w3772:dbl)
                n2210 = local read "N sets should be saved (MCL)"() -> (w3775:dbl)
                n2211 = Build Array(w3772, w3764, w3766, w3766, w3766) -> (w3770:dbl[])
                n2212 = Build Array(w3787, w3782, w3780, w3778, w3777, w3768, w3767) -> (w3784:dbl[])
                n2213 = Build Array(w3769, w3773, w3793, w3792, w3791, 3.0 ("t")) -> (w3786:dbl[])
                n2214 = Round Toward +Infinity(x=w3775) -> (ceil(x): smallest int >= x=w3776:dbl)
                n2215 = Build Array (concatenate)(w3786, w3785, w3770, w3784) -> (w3783:dbl[])
                n2216 = To Unsigned Long Integer(number=w3776) -> (unsigned 32bit integer=w3774:u32)
              }
            }
            n2217 = local read "Index"() -> (w3633:dbl)
            n2218 = call "Create new save file.vi"("Insert"="", "Ext"=".dat", "Index In"=w3633) -> ("Path Out"=w3592:path, "Index Out"=w3605:dbl)
            n2219 = local write "Save file name"(w3592) -> ()
            n2220 = local write "Index"(w3605) -> ()
            n2221 = local write "Save index"(w3605) -> ()
            n2222 = Array Size(array=w3616) -> (size(s)=w3617:i32)
            n2223 = Open/Create/Replace File(file path (use dialog)=w3592, operation (0:open)=T24."create", access (0:read/write)=enum16{"read/write", "read-only", "write-only"}."write-only") -> (refnum out=w3630:refnum<file>)  [unwired: 1 in, 4 out]
            n2224 = local write "Saving..."(TRUE ("Saving...")) -> ()
            n2225 = To Double Precision Float(number=w3617) -> (double precision float=w3615:dbl)
            n2226 = String Length(string="Comment (data description)") -> (length=w3613:i32)
            n2227 = To Double Precision Float(number=w3613) -> (double precision float=w3612:dbl)
            n2228 = Deny Access(7:w3630) -> (3:w3629:refnum<file>)  [unwired: 1 in, 2 out]
            n2229 = Build Array (concatenate)(w3615, w3616, w3612) -> (w3614:dbl[])
            n2230 = case "If fluorescence data to be saved" shown="True" w3603 {
              tunnel: w3592 -> [_ w3682]
              tunnel: [refnum<k0> refnum w3662] -> w3604
              frame False {
              }
              frame True {
                w3661 = 0.0
                n2231 = local read "APD Integration Time (s)"() -> (w3667:dbl)
                n2232 = local read "N APD Samp/step"() -> (w3660:dbl)
                n2233 = Path To String(path=w3682) -> (string=w3681:string)
                n2234 = String Length(string=w3681) -> (length=w3680:i32)
                n2235 = Subtract(x=w3680, y=4) -> (x-y=w3678:i32)
                n2236 = String Subset(string=w3681, length (rest)=w3678) -> (substring=w3677:string)  [unwired: 1 out]
                n2237 = Build Array(w3667, w3660, w3661, w3661, w3661, w3661, w3661, w3661) -> (w3664:dbl[])
                n2238 = Concatenate Strings(w3677, "_fl.dat" ("string")) -> (w3675:string)
                n2239 = Array Size(array=w3664) -> (size(s)=w3666:i32)
                n2240 = String To Path(string=w3675) -> (path=w3671:path)
                n2241 = Open/Create/Replace File(file path (use dialog)=w3671, operation (0:open)=T24."create", access (0:read/write)=enum16{"read/write", "read-only", "write-only"}."write-only") -> (refnum out=w3672:refnum<file>)  [unwired: 1 in, 4 out]
                n2242 = Deny Access(7:w3672) -> (3:w3668:refnum<file>)  [unwired: 1 in, 2 out]
                n2243 = To Double Precision Float(number=w3666) -> (double precision float=w3665:dbl)
                n2244 = Build Array (concatenate)(w3665, w3664) -> (w3663:dbl[])
                n2245 = Write to Binary File(file (use dialog)=w3668, data=w3663, 5:FALSE ("prepend array or string size? (T)"), 9:T30."big-endian, network order" ("byte order (0:big-endian, network order)")) -> (refnum out=w3662:refnum<file>)  [unwired: 1 in, 3 out]
              }
            }
            n2246 = case shown="True" w3590 {
              tunnel: w3592 -> [_ w3644]
              tunnel: [refnum<k0> refnum w3643] -> w3591
              frame False {
              }
              frame True {
                w3639 = 0.0 ("element")
                n2247 = Path To String(path=w3644) -> (string=w3658:string)
                n2248 = Build Array(w3639, w3639, w3639, w3639, w3639, w3639, w3639, w3639) -> (w3640:dbl[])
                n2249 = String Length(string=w3658) -> (length=w3657:i32)
                n2250 = Subtract(x=w3657, y=4) -> (x-y=w3655:i32)
                n2251 = Array Size(array=w3640) -> (size(s)=w3642:i32)
                n2252 = String Subset(string=w3658, length (rest)=w3655) -> (substring=w3654:string)  [unwired: 1 out]
                n2253 = To Double Precision Float(number=w3642) -> (double precision float=w3641:dbl)
                n2254 = Concatenate Strings(w3654, "_pos.dat" ("string")) -> (w3652:string)
                n2255 = Build Array (concatenate)(w3641, w3640) -> (w3638:dbl[])
                n2256 = String To Path(string=w3652) -> (path=w3648:path)
                n2257 = Open/Create/Replace File(file path (use dialog)=w3648, operation (0:open)=T24."create", access (0:read/write)=enum16{"read/write", "read-only", "write-only"}."write-only") -> (refnum out=w3649:refnum<file>)  [unwired: 1 in, 4 out]
                n2258 = Deny Access(7:w3649) -> (3:w3645:refnum<file>)  [unwired: 1 in, 2 out]
                n2259 = Write to Binary File(file (use dialog)=w3645, data=w3638, 5:FALSE ("prepend array or string size? (T)"), 9:T30."big-endian, network order" ("byte order (0:big-endian, network order)")) -> (refnum out=w3643:refnum<file>)  [unwired: 1 in, 3 out]
              }
            }
            n2260 = Write to Binary File(file (use dialog)=w3629, data=w3614, 5:w3610, 9:w3608) -> (refnum out=w3611:refnum<file>)  [unwired: 1 in, 3 out]
            n2261 = Write to Binary File(file (use dialog)=w3611, data="Comment (data description)", 5:w3610, 9:w3608) -> (refnum out=w3607:refnum<file>)  [unwired: 1 in, 3 out]
          }
        }
        n2262 = feedback-in #19(w3550) -> ()
        n2263 = feedback-in #20(w3577) -> ()
        n2264 = feedback-in #21(w3549) -> ()
        n2265 = feedback-in #22(w3560) -> ()
        n2266 = feedback-in #23(w3563) -> ()
        n2267 = feedback-in #24(w3576) -> ()
        n2268 = feedback-in #25(w3566) -> ()
      }
      frame #1 {
        n2269 = local read "Saving..."() -> (w3807:bool)
        n2270 = case shown="True" w3807 {
          tunnel: w3811 -> [_ w3821]
          tunnel: w3810 -> [_ w3835]
          tunnel: w3809 -> [_ w3831]
          tunnel: w3808 -> [_ w3830]
          tunnel: w3806 -> [_ w3829]
          tunnel: w3805 -> [_ w3824]
          tunnel: w3804 -> [_ w3823]
          tunnel: w3803 -> [_ w3822]
          tunnel: w3802 -> [_ w3820]
          tunnel: w3801 -> [_ w3818]
          tunnel: w3800 -> [_ w3817]
          tunnel: w3799 -> [_ w3816]
          tunnel: w3798 -> [_ w3815]
          tunnel: w3797 -> [_ w3814]
          tunnel: w3796 -> [_ w3813]
          tunnel: w3795 -> [_ w3812]
          frame False {
          }
          frame True {
            n2271 = Multiply(x=w3821, y=w3820) -> (x*y=→"Time (s)":dbl)
            n2272 = Less Or Equal?(x=w3821, y=w3829) -> (x <= y?=w3833:bool)
            n2273 = Or(x="Stop Saving", y="Abort save 2") -> (x .or. y?=w3825:bool)
            n2274 = Not(x=w3825) -> (.not. x?=w3834:bool)
            n2275 = And(x=w3833, y=w3834) -> (x .and. y?=w3832:bool)
            n2276 = case shown="True" w3832 {
              tunnel: w3835 -> [w3842 w3910]
              tunnel: [0.0 w3913] -> w3828
              tunnel: w3821 -> [_ w3911]
              tunnel: w3829 -> [_ w3912]
              tunnel: w3831 -> [_ w3907]
              tunnel: w3830 -> [_ _]
              tunnel: w3824 -> [w3840 w3900]
              tunnel: w3823 -> [w3839 w3901]
              tunnel: w3822 -> [_ w3899]
              tunnel: w3818 -> [_ w3898]
              tunnel: w3817 -> [_ w3852]
              tunnel: w3816 -> [_ w3891]
              tunnel: w3815 -> [_ w3869]
              tunnel: w3814 -> [w3837 w3850]
              tunnel: w3813 -> [w3838 w3849]
              tunnel: w3812 -> [_ w3846]
              frame False {
                w3836 = FALSE
                n2277 = Close File(refnum=w3842) -> ()  [unwired: 1 in, 2 out]
                n2278 = case shown="True" w3839 {
                  tunnel: w3840 -> [_ w3844]
                  frame False {
                  }
                  frame True {
                    n2279 = Close File(refnum=w3844) -> ()  [unwired: 1 in, 2 out]
                  }
                }
                n2280 = case shown="True" w3837 {
                  tunnel: w3838 -> [_ w3843]
                  frame False {
                  }
                  frame True {
                    n2281 = Close File(refnum=w3843) -> ()  [unwired: 1 in, 2 out]
                  }
                }
                n2282 = local write "Calibrating Trap..."(w3836) -> ()
                n2283 = call <vilib>:"Beep.vi"() -> ()  [unwired: 3 in, 9 out]
                n2284 = local write "Stop Saving"(w3836) -> ()
                n2285 = property on="Raster Scanning..." class="Bool (strict)"("Val(Sgnl)"=w3836) -> ()  [unwired: 2 in, 2 out]
                "Saving..." <- w3836
              }
              frame True {
                n2286 = local read "Calibrating Trap..."() -> (w3902:bool)
                n2287 = case "Write fl. data" shown="True" w3901 {
                  tunnel: w3900 -> [_ w3936]
                  tunnel: w3899 -> [_ w3935]
                  frame False {
                  }
                  frame True {
                    n2288 = Write to Binary File(file (use dialog)=w3936, data=w3935, 5:FALSE ("prepend array or string size? (T)"), 9:T30."big-endian, network order" ("byte order (0:big-endian, network order)")) -> ()  [unwired: 1 in, 4 out]
                  }
                }
                n2289 = Greater?(x="Save ave N", y=1.0) -> (0:w3905:bool)
                n2290 = Not(x=w3902) -> (.not. x?=w3904:bool)
                n2291 = And(x=w3904, y=w3905) -> (x .and. y?=w3847:bool)
                n2292 = case shown="True" w3847 {
                  tunnel: w3846 -> [w3916 w3927]
                  tunnel: [w3916 w3919] -> w3845
                  tunnel: "Save ave N" -> [_ w3920]
                  frame False {
                  }
                  frame True {
                    w3917 = 2 ("dimension size")
                    n2293 = Array Size(array=w3927) -> (size(s)=w3921:i32)
                    n2294 = Divide(x=w3921, y=w3917) -> (x/y=w3925:dbl)
                    n2295 = Reshape Array(w3927, w3925, w3917) -> (w3926:u64[][])
                    n2296 = Transpose 2D Array(2D array=w3926) -> (transposed array=w3924:u64[][])
                    n2297 = for {
                      tunnel: w3924 -> [w3929] mode=indexing
                      tunnel: [w3928] -> w3918 mode=indexing
                      tunnel: w3920 -> [w3930]
                      workers-P: _ -> [_]
                      n2298 = call "downsample 1D array - U64.vi"("Ave N"=w3930, "Array In"=w3929) -> ("Array Out"=w3928:u64[])  [unwired: 1 in]
                    }
                    n2299 = Transpose 2D Array(2D array=w3918) -> (transposed array=w3923:u64[][])
                    n2300 = Divide(x=w3921, y=w3920) -> (x/y=w3922:dbl)
                    n2301 = Reshape Array(w3923, w3922) -> (w3919:u64[])
                  }
                }
                n2302 = case shown="True" w3847 {
                  tunnel: w3907 -> [w3939 w3951]
                  tunnel: [w3939 w3943] -> w3903
                  tunnel: "Save ave N" -> [_ w3944]
                  tunnel: w3898 -> [_ w3942]
                  frame False {
                    # "don't downsample data for trap calibration"
                  }
                  frame True {
                    n2303 = Array Size(array=w3951) -> (size(s)=w3945:i32)
                    n2304 = Array Size(array=w3942) -> (size(s)=w3941:i32)
                    n2305 = Divide(x=w3945, y=w3941) -> (x/y=w3949:dbl)
                    n2306 = Reshape Array(w3951, w3949, w3941) -> (w3950:i16[][])
                    n2307 = Transpose 2D Array(2D array=w3950) -> (transposed array=w3948:i16[][])
                    n2308 = for {
                      tunnel: w3948 -> [w3954] mode=indexing
                      tunnel: [w3953] -> w3940 mode=indexing
                      tunnel: w3944 -> [w3952]
                      workers-P: _ -> [_]
                      n2309 = call "downsample 1D array - I16.vi"("Ave N"=w3952, "Array In"=w3954) -> ("Array Out"=w3953:i16[])  [unwired: 1 out]
                    }
                    n2310 = Transpose 2D Array(2D array=w3940) -> (transposed array=w3947:i16[][])
                    n2311 = Divide(x=w3945, y=w3944) -> (x/y=w3946:dbl)
                    n2312 = Reshape Array(w3947, w3946) -> (w3943:i16[])
                  }
                }
                n2313 = Index Array(array=w3869, index=1) -> (element=w3872:waveform(dbl))
                n2314 = Index Array(array=w3869, index=0) -> (element=w3874:waveform(dbl))
                n2315 = Unbundle By Name(w3872) -> ("Y"=w3876:dbl[])
                n2316 = Unbundle By Name(w3874) -> ("Y"=w3884:dbl[])
                n2317 = case "Write trap pos. data" shown="True" w3850 {
                  tunnel: w3849 -> [_ w3932]
                  tunnel: w3845 -> [_ w3931]
                  frame False {
                  }
                  frame True {
                    n2318 = Write to Binary File(file (use dialog)=w3932, data=w3931, 5:FALSE ("prepend array or string size? (T)"), 9:T30."big-endian, network order" ("byte order (0:big-endian, network order)")) -> ()  [unwired: 1 in, 4 out]
                  }
                }
